vi "Bi_lateralGalvoZStand_Analog.vi"(4 "stand Z vol Backward samp info":cluster{"Fs":dbl, "#s":dbl}={"Fs"=500000.0, "#s"=68421.0}, 6 "stand Z vol Acquisition samp info":cluster{"Fs":dbl, "#s":dbl}={"Fs"=500000.0, "#s"=131579.0}, 7 "Bi-lateral Galvo Z scan volt":dbl=0.45, 8 "error in (no error)":errorcluster, 9 "stand Z vol Backward time (s)":dbl=0.13684210526315793, 10 "Steps per volume":dbl=25.0, 11 "stand Z vol Acquisition time (s)":dbl=0.2631578947368421) -> (0 "error out":errorcluster, 3 "Bi-lateral Galvo Z stand":waveform(dbl))   [LabVIEW 2018]
panel:
  out "Preview":waveform(dbl)(graph)
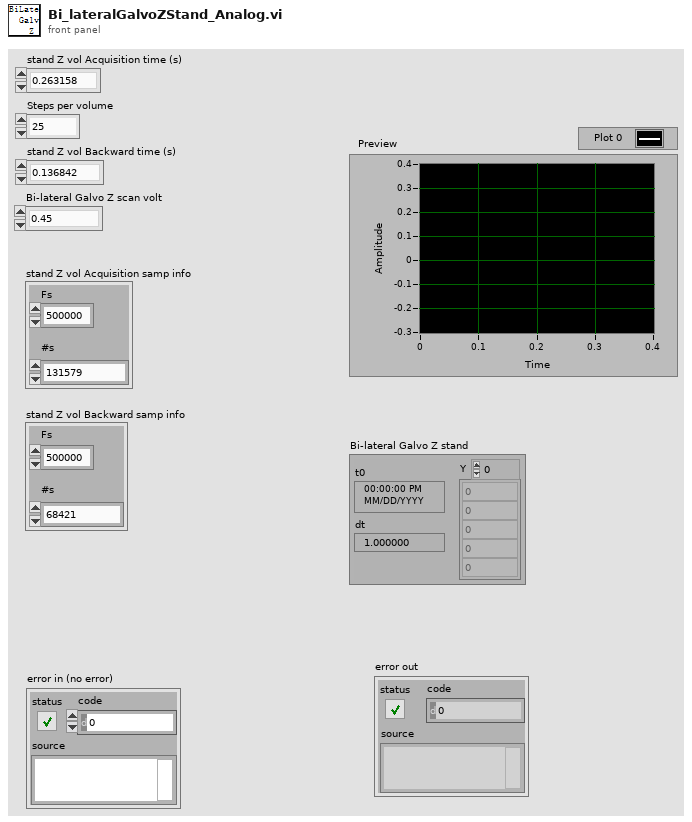
[diagram p1: front panel]
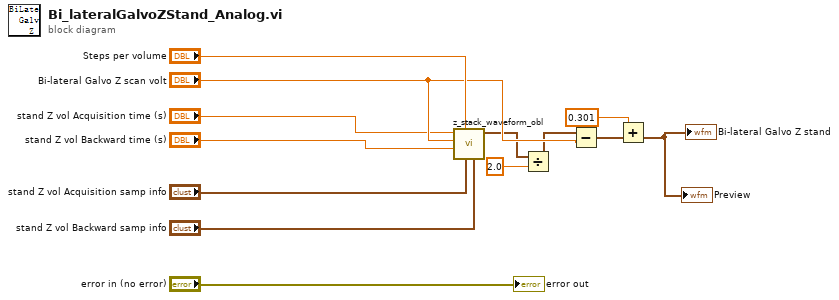
[diagram p0: block diagram]
diagram:
  n1 = call "z_stack_waveform_obl.vi"("Z stack backward"="stand Z vol Backward samp info", "Z stack acquisition"="stand Z vol Acquisition samp info", "Steps per Volume"="Steps per volume", "Backward Time (s)"="stand Z vol Backward time (s)", "SPECIFIC scan volt"="Bi-lateral Galvo Z scan volt", "Aquisition Time (s)"="stand Z vol Acquisition time (s)") -> ("WaveformOut"=w2:waveform(dbl))  [unwired: 5 in]
  n2 = Divide(x=w2, y=2.0) -> (x/y=w3:waveform(dbl))
  n3 = Subtract(x=w3, y="Bi-lateral Galvo Z scan volt") -> (x-y=w6:waveform(dbl))
  n4 = Add(x=0.301, y=w6) -> (x+y=→"Bi-lateral Galvo Z stand" →"Preview":waveform(dbl))
  "error out" <- "error in (no error)"
